vi "Parse Attribute.vi"(4 "Header Values":string[](array[string]), 6 "Header Names":string[](array[string]), 8 "error in (no error)":errorcluster, 9 "Tag Name":string, 10 "Flattened Linked List":string, 11 "CAML in":refnum<class "CAML.lvclass">) -> (0 "Error Out":errorcluster, 2 "Flattened Linked List out":string, 3 "CAML out":refnum<class "CAML.lvclass">, 5 "Attribute Value":variant, 7 "Attribute Name":string)   [LabVIEW 2020, in "CAML.lvlib" / "CAML.lvclass"]
uses:
  <vilib>/gpm_packages/@cs/persistence/source/CAML/CAML.lvclass
  <vilib>/Utility/error.llb/Error Cluster From Error Code.vi
  <vilib>/ErrorRing/Error Ring.xnode
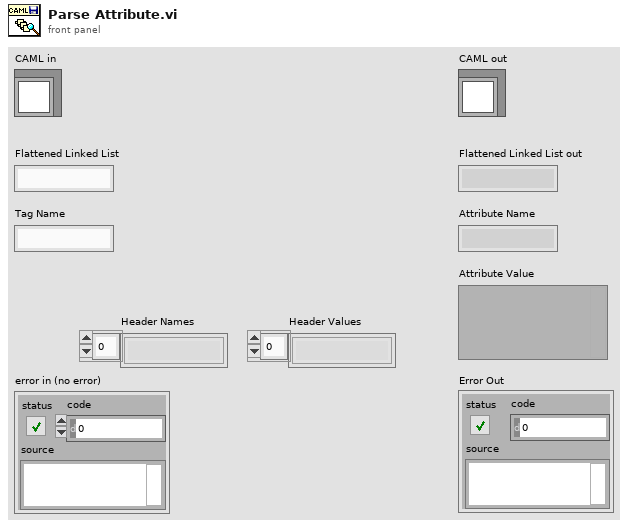
[diagram p1: front panel]
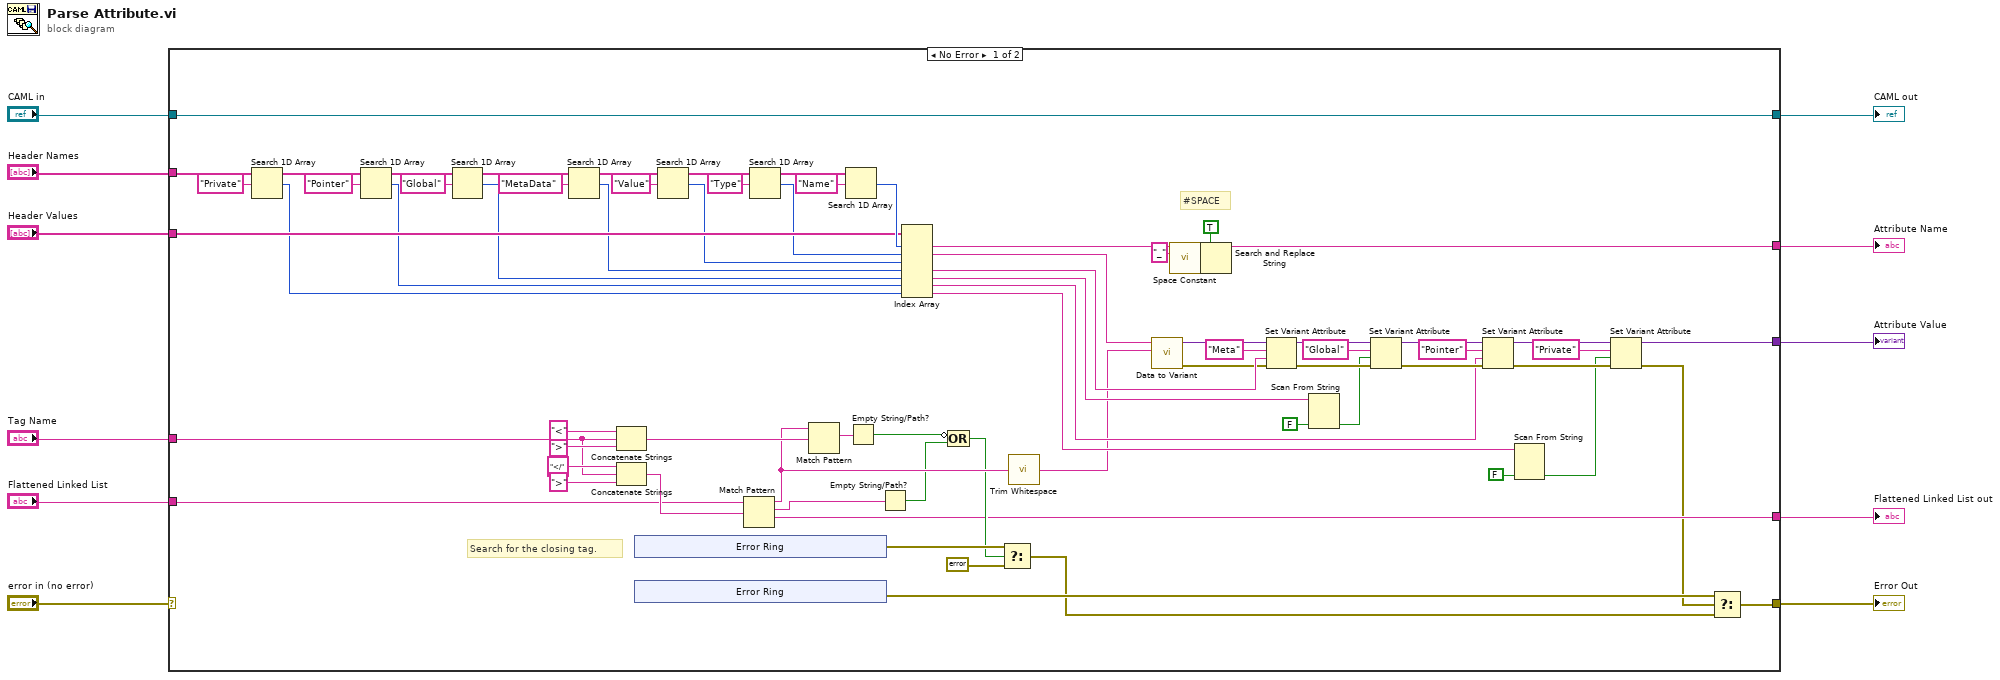
[diagram p0: block diagram]
diagram:
  n1 = case shown="No Error" "error in (no error)" {
    selector: "error in (no error)" -> [_ w88]
    tunnel: "CAML in" -> [w58 w90]
    tunnel: "Flattened Linked List" -> [w64 w89]
    tunnel: [w63 w89] -> w3
    tunnel: [w51 _] -> w1
    tunnel: [w21 _] -> w2
    tunnel: [w60 w88] -> w4
    tunnel: [w58 w90] -> w10
    tunnel: "Header Names" -> [w25 _]
    tunnel: "Header Values" -> [w55 _]
    tunnel: "Tag Name" -> [w54 _]
    frame No Error {
      # "#SPACE"
      # "Search for the closing tag."
      n2 = Search 1D Array(1D array=w25, element="Private") -> (index of element=w24:i32)  [unwired: 1 in]
      n3 = Search 1D Array(1D array=w25, element="Pointer") -> (index of element=w39:i32)  [unwired: 1 in]
      n4 = Search 1D Array(1D array=w25, element="Global") -> (index of element=w40:i32)  [unwired: 1 in]
      n5 = Search 1D Array(1D array=w25, element="MetaData") -> (index of element=w41:i32)  [unwired: 1 in]
      n6 = Concatenate Strings("<" ("string"), w54, ">" ("string")) -> (w70:string)
      n7 = Concatenate Strings("</" ("string"), w54, ">" ("string")) -> (w73:string)
      n8 = xnode "Error Ring"() -> ("error out"=w76:errorcluster)
      n9 = xnode "Error Ring"() -> ("error out"=w62:errorcluster)
      n10 = Search 1D Array(1D array=w25, element="Value") -> (index of element=w42:i32)  [unwired: 1 in]
      n11 = Match Pattern(string=w64, regular expression=w73) -> (before substring=w69:string, match substring=w77:string, after substring=w63:string)  [unwired: 1 in, 1 out]
      n12 = Search 1D Array(1D array=w25, element="Type") -> (index of element=w43:i32)  [unwired: 1 in]
      n13 = Match Pattern(string=w69, regular expression=w70) -> (match substring=w68:string)  [unwired: 1 in, 3 out]
      n14 = Search 1D Array(1D array=w25, element="Name") -> (index of element=w56:i32)  [unwired: 1 in]
      n15 = Empty String/Path?(string/path=w68) -> (empty?=w67:bool)
      n16 = Empty String/Path?(string/path=w77) -> (empty?=w66:bool)
      n17 = Index Array(array=w55, index #1=w56, index #2=w43, index #3=w42, index #4=w41, index #5=w40, index #6=w39, index #7=w24) -> (element #1=w52:string, element #2=w15:string, element #4=w35:string, element #5=w28:string, element #6=w27:string, element #7=w17:string)  [unwired: 1 out]
      n18 = Compound Arithmetic op=OR(invert w67, w66) -> (w65:bool)
      n19 = Select(t=w76, s=w65, f=errorcluster {"status"=FALSE, "code"=0, "source"=""}) -> (s? t:f=w59:errorcluster)
      n20 = call <vilib>:"Trim Whitespace.vi"("string"=w69) -> ("trimmed string"=w14:string)  [unwired: 1 in]
      n21 = call <vilib>:"Data to Variant.vi"("Value"=w14, "Type"=w15) -> ("error out"=w12:errorcluster, "Variant"=w13:variant)  [unwired: 8 in]
      n22 = call <vilib>:"Space Constant.vi"() -> ("String"=w49:string)
      n23 = Search and Replace String(replace all?=TRUE ("replace all? (F)"), input string=w52, search string="_", replace string=w49) -> (result string=w51:string)  [unwired: 4 in, 3 out]
      n24 = Set Variant Attribute(Variant=w13, name="Meta", value=w35, error in=w12) -> (Variant out=w38:variant, error out=w33:errorcluster)  [unwired: 1 out]
      n25 = Scan From String(input string=w28, default 1=FALSE) -> (output 1=w31:bool)  [unwired: 3 in, 3 out]
      n26 = Set Variant Attribute(Variant=w38, name="Global", value=w31, error in=w33) -> (Variant out=w37:variant, error out=w29:errorcluster)  [unwired: 1 out]
      n27 = Set Variant Attribute(Variant=w37, name="Pointer", value=w27, error in=w29) -> (Variant out=w22:variant, error out=w20:errorcluster)  [unwired: 1 out]
      n28 = Scan From String(input string=w17, default 1=FALSE) -> (output 1=w16:bool)  [unwired: 3 in, 3 out]
      n29 = Set Variant Attribute(Variant=w22, name="Private", value=w16, error in=w20) -> (Variant out=w21:variant, error out=w19:errorcluster)  [unwired: 1 out]
      n30 = Select(t=w62, s=w19, f=w59) -> (s? t:f=w60:errorcluster)
    }
    frame Error {
    }
  }
  "CAML out" <- w10
  "Flattened Linked List out" <- w3
  "Attribute Name" <- w1
  "Attribute Value" <- w2
  "Error Out" <- w4
